vi "create Score.vi"(8 "error in (no error)":errorcluster, 10 "Score":u32, 11 "Score in":refnum<class "Score.lvclass">) -> (0 "error out":errorcluster, 3 "Score out":refnum<class "Score.lvclass">)   [LabVIEW 2019, in "Score.lvclass"]
uses:
  Score.lvclass
  TCP Packet/Packet.lvclass
  TCP Packet/packet type STYP.ctl
  C:/projects/labview_multiplayer_snake/Main Codeline/Software/Code/Shared/TCP Packet/Packet.lvclass
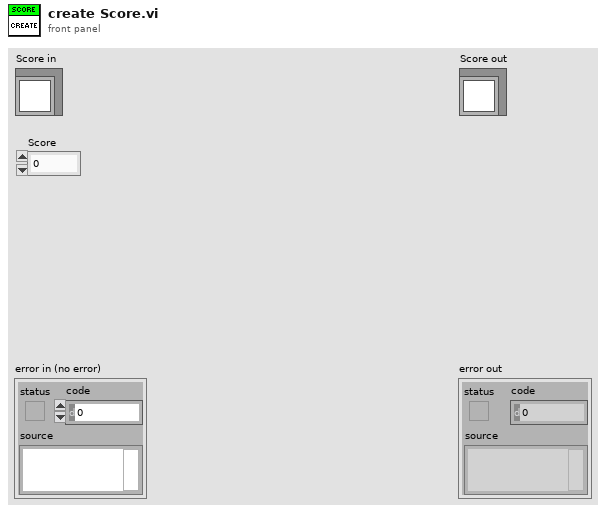
[diagram p1: front panel]
types:
  T1 = typedef "Packet.lvclass/packet type STYP.ctl" = enum16{"Connect", "Disconnect", "Direction", "Score", "Map"}
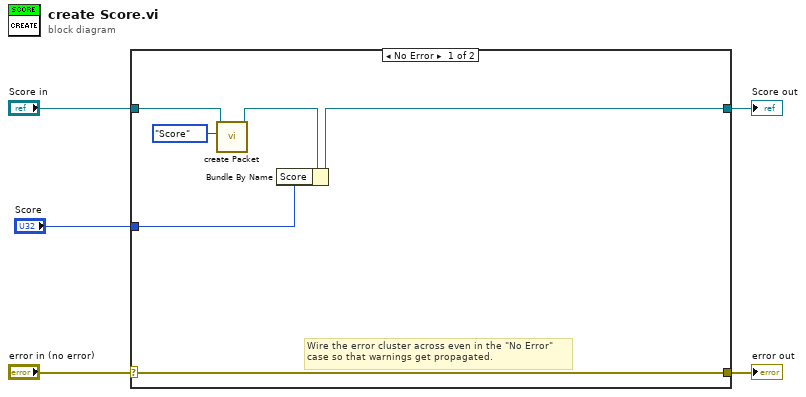
[diagram p0: block diagram]
diagram:
  n1 = case shown="No Error" "error in (no error)" {
    selector: "error in (no error)" -> [w11 w13]
    tunnel: [w11 w13] -> w4
    tunnel: [w7 w12] -> w2
    tunnel: "Score in" -> [w9 w12]
    tunnel: "Score" -> [w6 _]
    frame No Error {
      # "Wire the error cluster across even in the \"No Error\"\ncase so that warnings get propagated."
      n2 = call "create Packet.vi"("Packet Type"=packet_type_STYP."Score", "Packet in"=w9) -> ("Packet out"=w10:refnum<class "Score.lvclass">)  [unwired: 8 in, 1 out]
      n3 = Bundle By Name(cluster=w10, "Score"=w6) -> (w7:refnum<class "Score.lvclass">)
    }
    frame Error {
    }
  }
  "error out" <- w4
  "Score out" <- w2
